vi "Valco - Close.vi"(11 "VISA resource name":refnum<visa-resource-name>="COM3") -> (0 "error out":errorcluster)   [LabVIEW 2018]
panel:
  out "read buffer":string
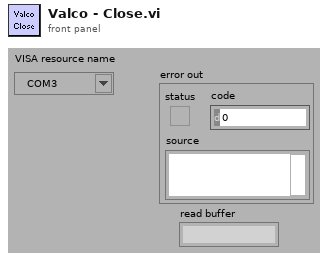
[diagram p1: front panel]
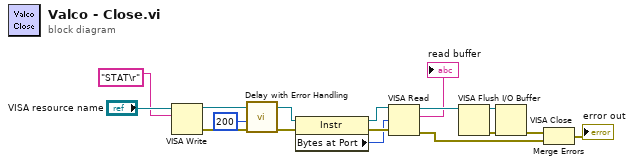
[diagram p0: block diagram]
diagram:
  n1 = VISA Write(VISA resource name="VISA resource name", write buffer="STAT\r" ("string")) -> (VISA resource name out=w6:refnum<visa-resource-name>, error out=w8:errorcluster)  [unwired: 1 in, 1 out]
  n2 = call "Delay with Error Handling.vi"("error in (no error)"=w8, "Delay (ms)"=u32 200) -> ("error out"=w2:errorcluster)  [unwired: 9 in]
  n3 = property class="Instr"(reference=w6, error in=w2) -> (reference out=w5:refnum<visa-resource-name>, error out=w7:errorcluster, "Bytes at Port"=w4:u32)
  n4 = VISA Read(VISA resource name=w5, byte count=w4, error in (no error)=w7) -> (VISA resource name out=w11:refnum<visa-resource-name>, read buffer=→"read buffer":string, error out=w9:errorcluster)  [unwired: 1 out]
  n5 = VISA Flush I/O Buffer(VISA resource name=w11) -> (VISA resource name out=w15:refnum<visa-resource-name>, error out=w14:errorcluster)  [unwired: 2 in]
  n6 = VISA Close(VISA resource name=w15, error in (no error)=w14) -> (error out=w16:errorcluster)
  n7 = Merge Errors(w16, w9) -> (→"error out":errorcluster)
